vi "Read Custom SCP Commands List Property.vi"(6 "Add 1st Column Idx? (T)":bool=TRUE, 8 "error in (no error)":errorcluster, 11 "Node Ptr":T1 format="%.0x") -> (0 "error out":errorcluster, 2 "Custom SCP Commands List":string[][](array[string]), 3 "Item Ref out":T1 format="%.0x")   [LabVIEW 2023, in "Vires VTD System Explorer.lvlib"]
doc: "Reads 2D array of strings to CD Item Property and adds first column with item index"
uses:
  Vires VTD System Explorer.lvlib
  <vilib>/NI VeriStand/Custom Device API/Custom Device Item Ref.ctl
  Shared/Constants.vi
  <vilib>/NI VeriStand/Custom Device API/Get Item Property (Variant).vi
  <vilib>/NI VeriStand/Custom Device API/Custom Device API.lvlib
  Shared/Vires VTD Shared.lvlib
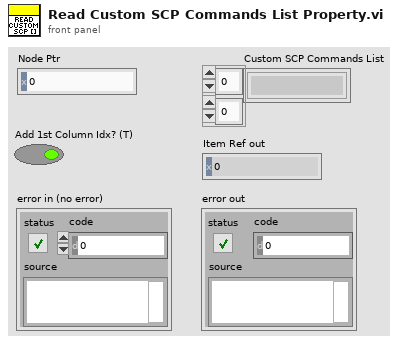
[diagram p1: front panel]
types:
  T1 = typedef "Custom Device API.lvlib/Custom Device Item Ref.ctl" = u64
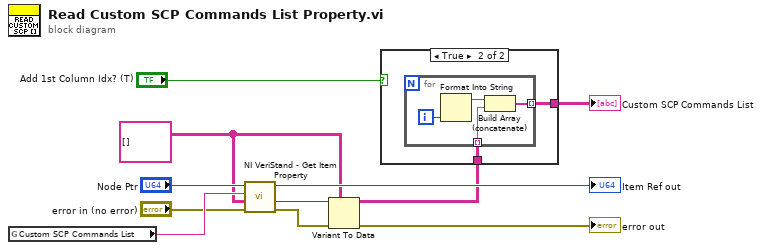
[diagram p0: block diagram]
diagram:
  w3 = string[][] [] ("Default Value")
  n1 = global read "Constants.vi" "Custom SCP Commands List"() -> (w11:string)
  n2 = call-poly <vilib>:"NI VeriStand - Get Item Property.vi"("error in (no error)"="error in (no error)", "Default Value"=w3, "Property Name"=w11, "Item Ref in"="Node Ptr") -> ("error out"=w5:errorcluster, "Value"=w6:variant, "Item Ref out"=→"Item Ref out":T1)  [unwired: 4 in, 1 out]
  n3 = Variant To Data(error in=w5, type=w3, Variant=w6) -> (data=w2:string[][], error out=→"error out":errorcluster)
  n4 = case shown="True" "Add 1st Column Idx? (T)" {
    tunnel: [w12 w14] -> w10
    tunnel: w2 -> [w12 w13]
    frame False {
    }
    frame True {
      n5 = for {
        tunnel: w13 -> [w16] mode=indexing
        tunnel: [w15] -> w14 mode=indexing
        i -> [w18]
        n6 = Format Into String(w18) -> (resulting string=w17:string)  [unwired: 3 in, 1 out]
        n7 = Build Array (concatenate)(w17, w16) -> (w15:string[])
      }
    }
  }
  "Custom SCP Commands List" <- w10
